vi "I2C_ReadByteFromSlave_2.vi"(5 "InterByteTransmitDelay(Ticks)":u32, 7 "HalfCycle(Ticks)":u32, 8 "error in":errorcluster, 10 "StatusIn":i16, 11 "NumBytesToRead":i32) -> (0 "error out":errorcluster, 2 "Status":i16)   [LabVIEW 2019]
doc: "Reads the specified number of Data Bytes from the Slave Device & Transfers the Bytes into the Read memory block on the FPGA for the Host VI to access when the reading is complete.\n\n<b>Inputs:</b>\n---------------------\n<b>HalfCycle(Ticks)</b> this the number of FPGA clock cycles in half og the clock period. Therefore twice this number yields the clock period, in ticks.\n\n<b>InterByteTranmitDelay(Ticks)</b> the delay in FPGA clock cycles before writing the next byte on the SDA line.\n\n<b>NumBytesToRead</b> the number of bytes to read from the Slave Device.\n\n<b>StatusIn</b> the status of the Slave Device / I2C Bus\n\n<b>Outputs:</b>\n---------------------\n<b>Status</b> returns a numeric value representing the status of the I2C bus / slave device.\n0 = slave responded\n5002 = slave did not respond\n\nSee block diagram for more details on the implementation details.\n\nAuthor:\nPeter Fuller\nSenior Engineer\nPLF Consulting, LLC\n\nemail: peter@plfconsulting.com\nphone: 617.699.2201"
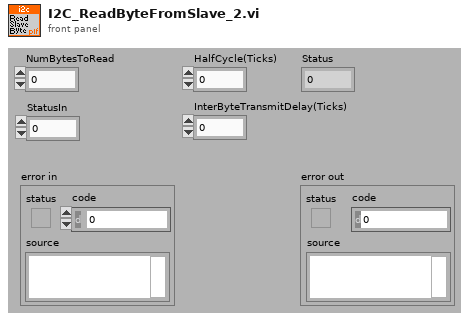
[diagram p1: front panel]
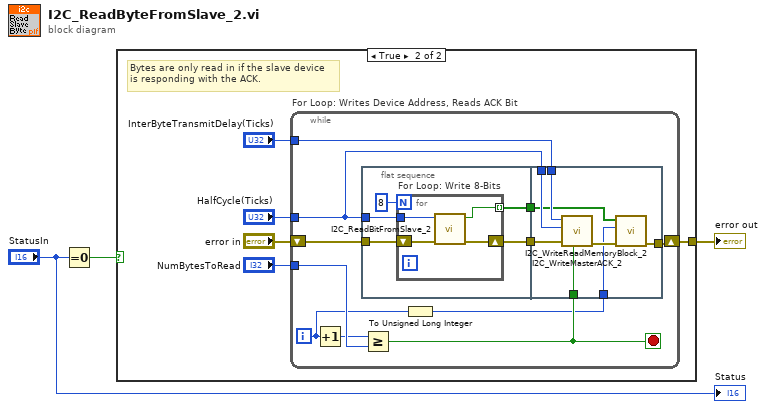
[diagram p0: block diagram]
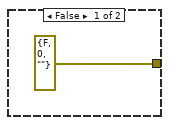
[diagram p2: hidden frame]
diagram:
  n1 = Equal To 0?(x="StatusIn") -> (x = 0?=w2:bool)
  n2 = case shown="True" w2 {
    tunnel: [errorcluster {"status"=FALSE, "code"=0, "source"=""} ("error in") w8] -> w3
    frame False {
    }
    frame True {
      # "Bytes are only read in if the slave device\nis responding with the ACK."
      n3 = while "For Loop: Writes Device Address, Reads ACK Bit" {
        tunnel: "HalfCycle(Ticks)" -> [w12]
        shift-right: [w10] -> w8
        shift-left: "error in" -> [w20]
        tunnel: "NumBytesToRead" -> [w17]
        tunnel: "InterByteTransmitDelay(Ticks)" -> [w13]
        i -> [w15]
        stop <- w14 stop-if-true
        n4 = Increment(x=w15) -> (x+1=w16:i32)
        n5 = flat-sequence {
          tunnel: w12 -> [w22]
          tunnel: w20 -> [w24]
          tunnel: [w23] -> w19
          tunnel: [w21] -> w18
          tunnel: w19 -> [w34]
          tunnel: w18 -> [w31]
          tunnel: w14 -> [w35]
          tunnel: w13 -> [w37]
          tunnel: w12 -> [w36]
          tunnel: w11 -> [w30]
          tunnel: [w32] -> w10
          frame #0 {
            n6 = for "For Loop: Write 8-Bits" {
              N: 8 -> [_]
              shift-right: [w26] -> w23
              shift-left: w24 -> [w27]
              tunnel: w22 -> [w29]
              tunnel: [w28] -> w21 mode=indexing
              n7 = call "I2C_ReadBitFromSlave_2.vi"("error in"=w27, "HalfCycle(Ticks)"=w29) -> ("error out"=w26:errorcluster, "Bit"=w28:bool)  [unwired: 8 in]
            }
          }
          frame #1 {
            n8 = call "I2C_WriteMasterACK_2.vi"("ACK"=w35, "error in"=w34, "HalfCycle(Ticks)"=w36, "InterByteTransmitDelay(Ticks)"=w37) -> ("error out"=w33:errorcluster)  [unwired: 6 in, 1 out]
            n9 = call "I2C_WriteReadMemoryBlock_2.vi"("error in (no error)"=w33, "MemoryAddress"=w30, "Bits"=w31) -> ("error out"=w32:errorcluster)  [unwired: 8 in]
          }
        }
        n10 = Greater Or Equal?(x=w16, y=w17) -> (x >= y?=w14:bool)
        n11 = To Unsigned Long Integer(number=w15) -> (unsigned 32bit integer=w11:u32)
      }
    }
  }
  "error out" <- w3
  "Status" <- "StatusIn"
